vi "Query Auto Save.vi"(8 "error IO":errorcluster, 11 "VISA resource name":refnum<visa-resource-name>) -> (0 "error Out":errorcluster, 2 "Auto Save?":bool, 3 "VISA resource Out":refnum<visa-resource-name>)   [LabVIEW 2020, in "eec EST 300.lvlib"]
doc: "Query the status of Auto Save enable or not."
uses:
  <instrlib>/eec EST 300/eec EST 300.lvlib
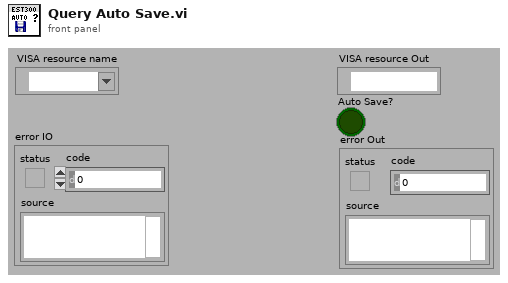
[diagram p1: front panel]
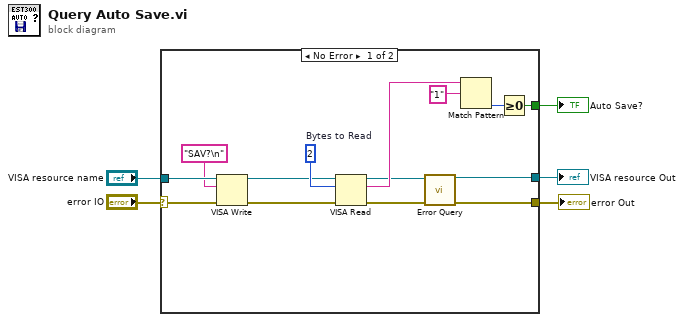
[diagram p0: block diagram]
diagram:
  n1 = case shown="No Error" "error IO" {
    selector: "error IO" -> [w19 w21]
    tunnel: [w16 w21] -> w1
    tunnel: [w17 w20] -> w3
    tunnel: "VISA resource name" -> [w18 w20]
    tunnel: [w12 _] -> w2
    frame No Error {
      w10 = u32 2  # Bytes to Read
      n2 = VISA Write(VISA resource name=w18, write buffer="SAV?\n" ("Command to Send (empty)"), error in (no error)=w19) -> (VISA resource name out=w7:refnum<visa-resource-name>, error out=w6:errorcluster)  [unwired: 1 out]
      n3 = VISA Read(VISA resource name=w7, byte count=w10, error in (no error)=w6) -> (VISA resource name out=w9:refnum<visa-resource-name>, read buffer=w11:string, error out=w8:errorcluster)  [unwired: 1 out]
      n4 = call <instrlib>:"Error Query.vi"("VISA resource name"=w9, "error in (no error)"=w8) -> ("VISA resource name out"=w17:refnum<visa-resource-name>, "error out"=w16:errorcluster)  [unwired: 10 in, 2 out]
      n5 = Match Pattern(string=w11, regular expression="1" ("search string")) -> (offset past match=w14:i32)  [unwired: 1 in, 3 out]
      n6 = Greater Or Equal To 0?(x=w14) -> (x >= 0?=w12:bool)
    }
    frame Error {
    }
  }
  "VISA resource Out" <- w3
  "Auto Save?" <- w2
  "error Out" <- w1
